vi "Control+sensors.vi"() -> ()   [LabVIEW 2025]
panel:
  in  "stop":bool
  out "String 2":string
  out "Boolean 5":bool
  out "Boolean 4":bool
  out "Boolean 3":bool
  out "Boolean 2":bool
  in  "Boolean":bool
  in  "Velocity":dbl(slide) scale=0.0..10.0
  in  "40":bool
  in  "70":bool
  in  "100":bool
  in  "Don't moove":bool
  in  "L":bool
  in  "D":bool
  in  "R":bool
  in  "U":bool
  # "IR Sensors"
  # "Manual"
  # "Auto"
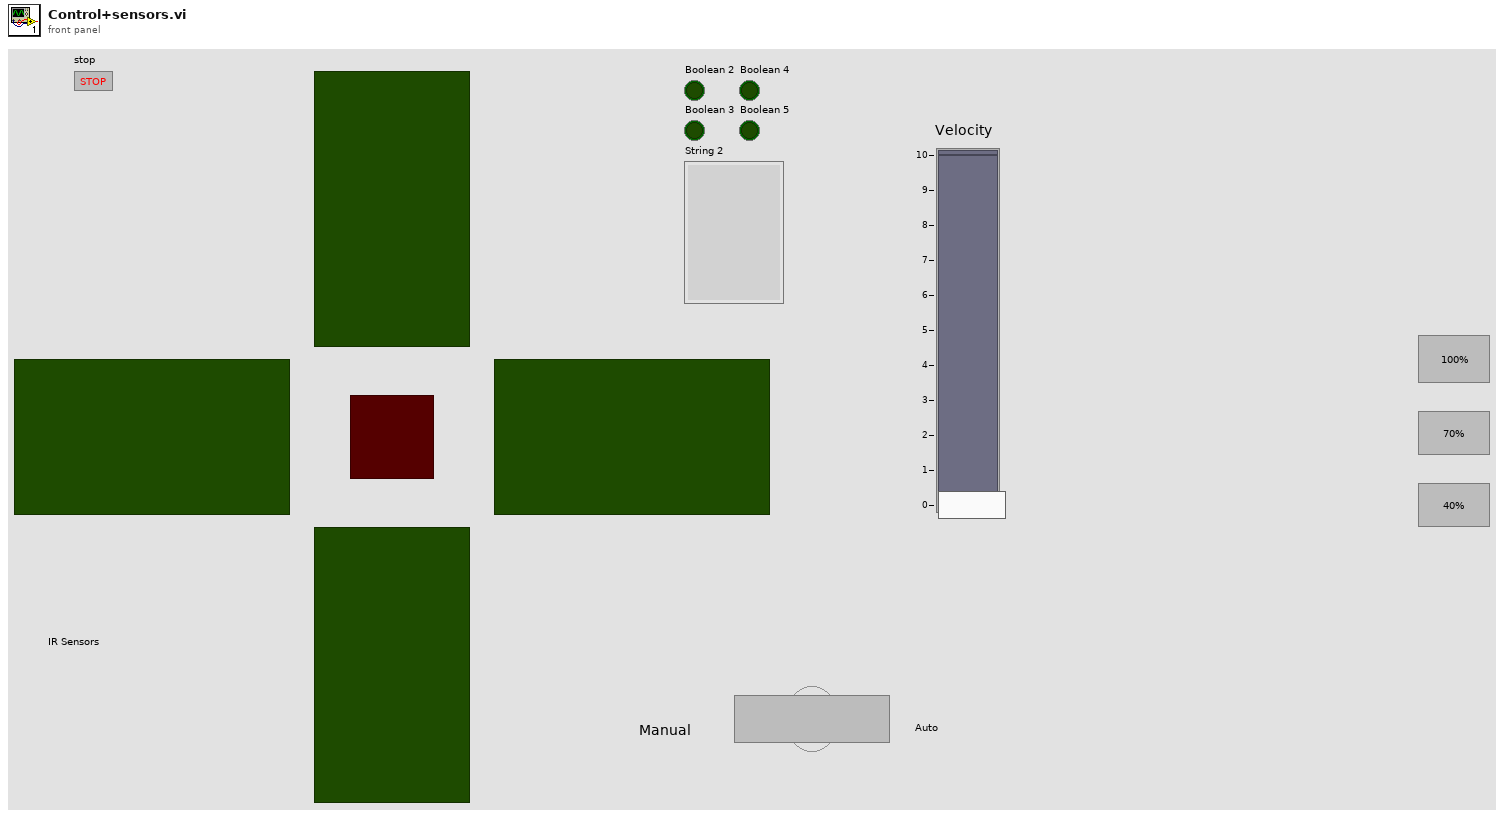
[diagram p1: front panel]
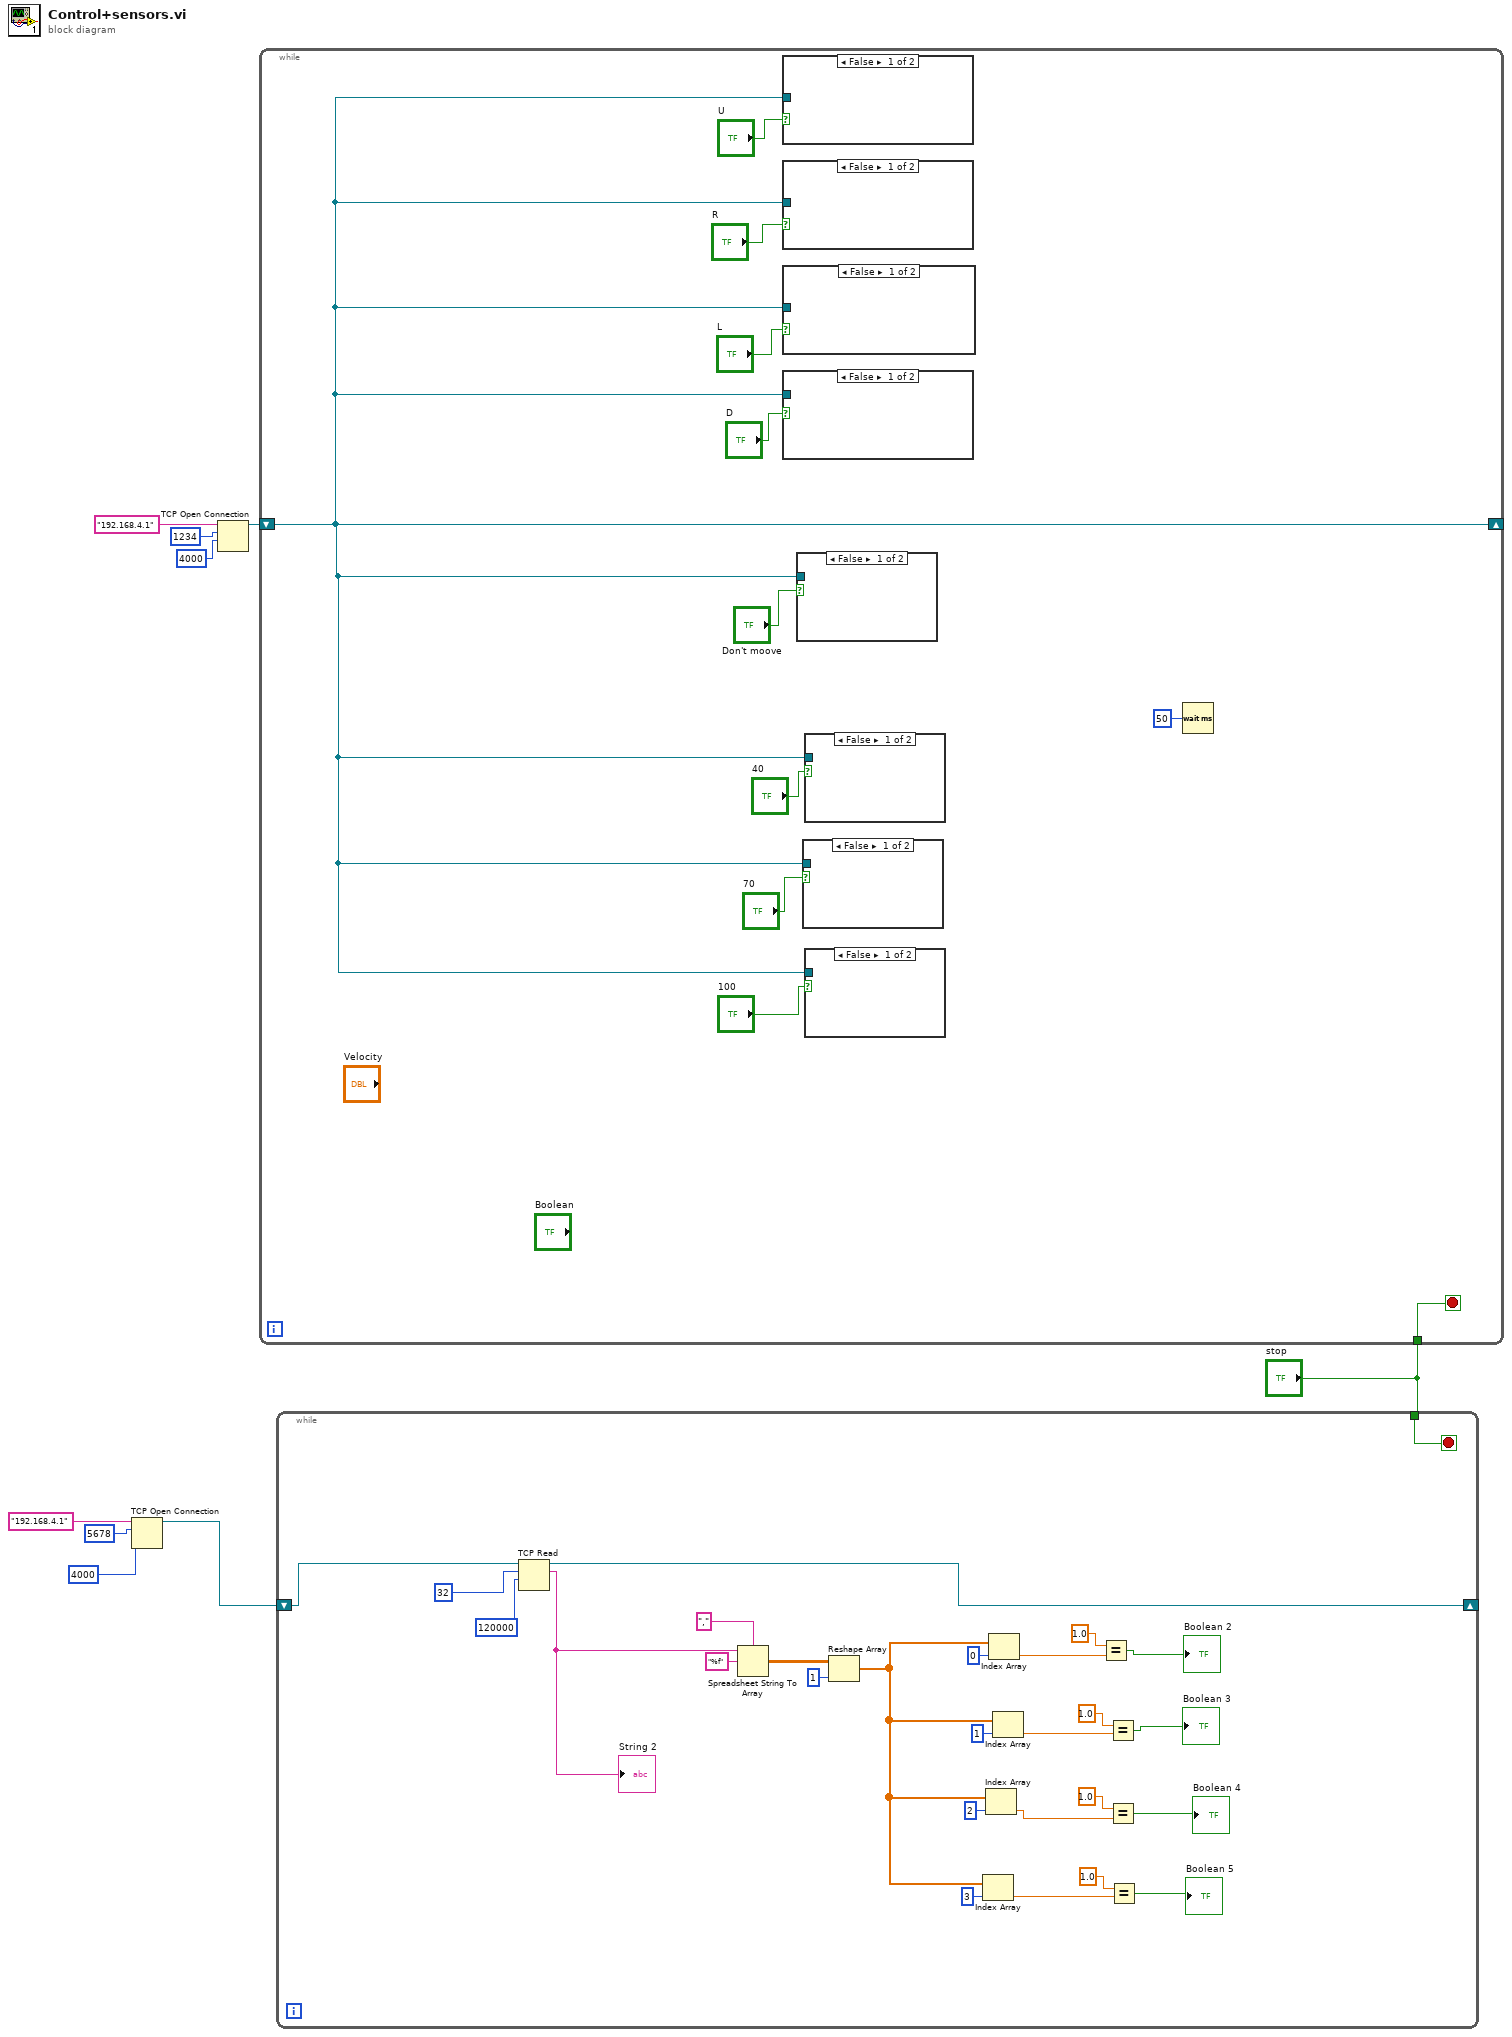
[diagram p0: block diagram]
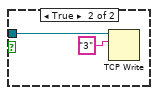
[diagram p2: hidden frame]
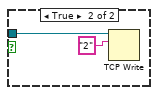
[diagram p3: hidden frame]
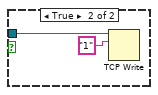
[diagram p4: hidden frame]
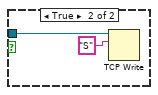
[diagram p5: hidden frame]
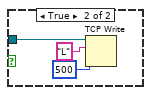
[diagram p6: hidden frame]
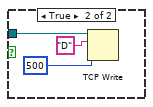
[diagram p7: hidden frame]
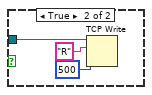
[diagram p8: hidden frame]
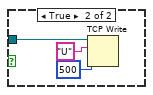
[diagram p9: hidden frame]
diagram:
  n1 = TCP Open Connection(address="192.168.4.1", remote port or service name=u16 5678, timeout ms (60000)=4000) -> (connection ID=w2:refnum<k5>)  [unwired: 2 in, 1 out]
  n2 = TCP Open Connection(address="192.168.4.1", remote port or service name=u16 1234, timeout ms (60000)=4000) -> (connection ID=w7:refnum<k5>)  [unwired: 2 in, 1 out]
  n3 = while {
    shift-right: [w11] -> _
    shift-left: w7 -> [w11]
    tunnel: "stop" -> [w10]
    stop <- w10 stop-if-true
    n4 = case shown="False" "U" {
      tunnel: w11 -> [_ w40]
      frame False {
      }
      frame True {
        n5 = TCP Write(connection ID=w40, data in="U", 9:500 ("timeout ms (25000)")) -> ()  [unwired: 1 in, 3 out]
      }
    }
    n6 = case shown="False" "R" {
      tunnel: w11 -> [_ w37]
      frame False {
      }
      frame True {
        n7 = TCP Write(connection ID=w37, data in="R", 9:500 ("timeout ms (25000)")) -> ()  [unwired: 1 in, 3 out]
      }
    }
    n8 = case shown="False" "L" {
      tunnel: w11 -> [_ w31]
      frame False {
      }
      frame True {
        n9 = TCP Write(connection ID=w31, data in="L", 9:500 ("timeout ms (25000)")) -> ()  [unwired: 1 in, 3 out]
      }
    }
    n10 = case shown="False" "D" {
      tunnel: w11 -> [_ w34]
      frame False {
      }
      frame True {
        n11 = TCP Write(connection ID=w34, data in="D", 9:500 ("timeout ms (25000)")) -> ()  [unwired: 1 in, 3 out]
      }
    }
    n12 = case shown="False" "Don't moove" {
      tunnel: w11 -> [_ w28]
      frame False {
      }
      frame True {
        n13 = TCP Write(connection ID=w28, data in="S") -> ()  [unwired: 2 in, 3 out]
      }
    }
    n14 = case shown="False" "70" {
      tunnel: w11 -> [_ w24]
      frame False {
      }
      frame True {
        n15 = TCP Write(connection ID=w24, data in="2") -> ()  [unwired: 2 in, 3 out]
      }
    }
    n16 = case shown="False" "40" {
      tunnel: w11 -> [_ w26]
      frame False {
      }
      frame True {
        n17 = TCP Write(connection ID=w26, data in="1") -> ()  [unwired: 2 in, 3 out]
      }
    }
    n18 = case shown="False" "100" {
      tunnel: w11 -> [_ w22]
      frame False {
      }
      frame True {
        n19 = TCP Write(connection ID=w22, data in="3") -> ()  [unwired: 2 in, 3 out]
      }
    }
    n20 = Wait (ms)(milliseconds to wait=u32 50) -> ()  [unwired: 1 out]
  }
  n21 = while {
    shift-right: [w42] -> _
    shift-left: w2 -> [w43]
    tunnel: "stop" -> [w41]
    stop <- w41 stop-if-true
    n22 = TCP Read(connection ID=w43, bytes to read=32, 9:120000 ("timeout ms (25000)")) -> (connection ID out=w42:refnum<k5>, data out=w46:string)  [unwired: 2 in, 1 out]
    "String 2" <- w46
    n23 = Spreadsheet String To Array(delimiter (Tab)=",", format string=w46, spreadsheet string="%f") -> (array=w67:dbl[][])  [unwired: 1 in]
    n24 = Reshape Array(w67, 1 ("dimension size")) -> (w64:dbl[])
    n25 = Index Array(array=w64, index=3) -> (element=w62:dbl)
    n26 = Index Array(array=w64, index=2) -> (element=w63:dbl)
    n27 = Index Array(array=w64, index=0) -> (element=w66:dbl)
    n28 = Index Array(array=w64, index=1) -> (element=w65:dbl)
    n29 = Equal?(x=1.0, y=w66) -> (x = y?=→"Boolean 2":bool)
    n30 = Equal?(x=1.0, y=w65) -> (x = y?=→"Boolean 3":bool)
    n31 = Equal?(x=1.0, y=w63) -> (x = y?=→"Boolean 4":bool)
    n32 = Equal?(x=1.0, y=w62) -> (x = y?=→"Boolean 5":bool)
  }
